vi "Current Capacitance Measurement E4990A.vi"(7 "RFFE In":refnum<visa-resource-name>, 8 "Error In":errorcluster, 10 "E4980A LCR In":refnum<visa-resource-name>, 11 "KE2000 In":refnum<visa-resource-name>) -> (0 "Error Out":errorcluster, 1 "uA":string, 2 "E4980A LCR Out":refnum<visa-resource-name>, 3 "KE2000 Out":refnum<visa-resource-name>, 4 "Cap(fF)":dbl, 5 "RFFE Out":refnum<visa-resource-name>)   [LabVIEW 2017]
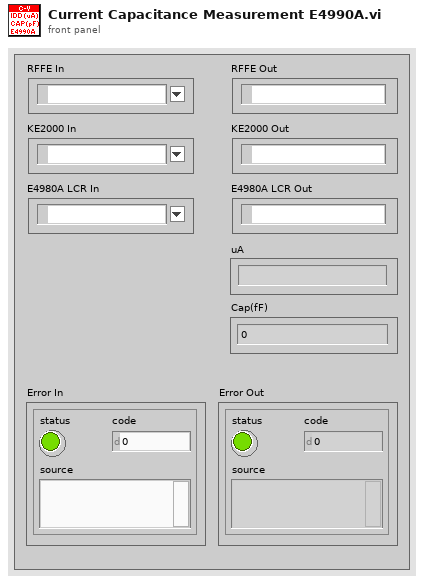
[diagram p1: front panel]
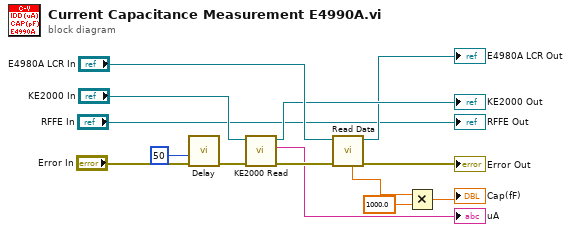
[diagram p0: block diagram]
diagram:
  n1 = call "Delay.vi"("error in (no error)"="Error In", "Delay"=u32 50) -> ("error out"=w13:errorcluster)  [unwired: 9 in]
  n2 = call "KE2000 Read.vi"("error in (no error)"=w13, "VISA resource name"="KE2000 In") -> ("error out"=w12:errorcluster, "uA"=→"uA":string, "VISA resource name out"=→"KE2000 Out":refnum<visa-resource-name>)  [unwired: 7 in]
  n3 = call "Read Data.vi"("Error In"=w12, "VISA IN"="E4980A LCR In") -> ("Error Out"=→"Error Out":errorcluster, "VISA Out"=→"E4980A LCR Out":refnum<visa-resource-name>, "CAP (pF)"=w4:dbl)  [unwired: 5 in, 2 out]
  n4 = Multiply(x=w4, y=1000.0) -> (x*y=→"Cap(fF)":dbl)
  "RFFE Out" <- "RFFE In"
